vi "testVI.vi"() -> ()   [LabVIEW 2015]
panel:
  out "Remote Call":bool
  out "result string":string
  out "VI Path 2":path
  out "call chain":string[](array[string])
  out "VI Path":path
  out "Is Clone VI":bool
  out "Is In Packed Library":bool
  out "Is Instance":bool
  out "Is Probe":bool
  out "Callers' Names":string[](array[string])
  out "Execution:Preferred Exec System":T1(ring)
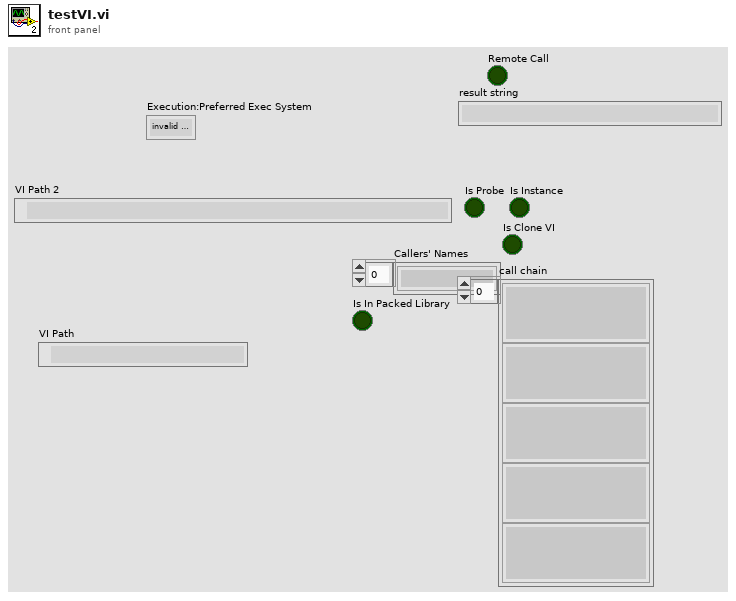
[diagram p1: front panel]
types:
  T1 = enum32{"invalid execution system", "user interface", "standard", "instrument i/o", "data acquisition", "other 1", "other 2", "same as caller"}
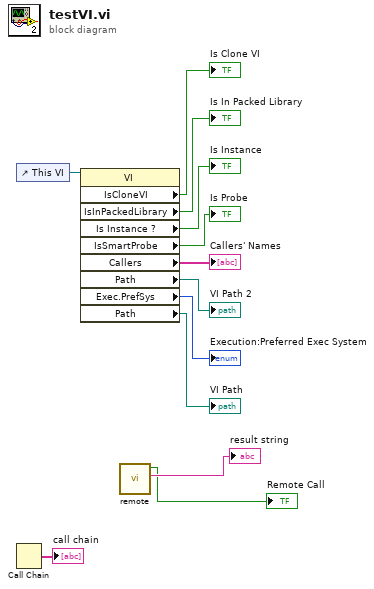
[diagram p0: block diagram]
diagram:
  n1 = Call Chain() -> (call chain=→"call chain":string[])
  n2 = control-ref of="This VI"() -> (w12:refnum<vi>)
  n3 = property class="VI"(reference=w12) -> ("IsCloneVI"=→"Is Clone VI":bool, "IsInPackedLibrary"=→"Is In Packed Library":bool, "Is Instance ?"=→"Is Instance":bool, "IsSmartProbe"=→"Is Probe":bool, "Callers"=→"Callers' Names":string[], "Path"=→"VI Path 2":path, "Exec.PrefSys"=→"Execution:Preferred Exec System":T1, "Path"=→"VI Path":path)  [unwired: 1 in, 2 out]
  n4 = call "remote.vi"() -> ("Caller string"=→"result string":string, "Remote Call"=→"Remote Call":bool)  [unwired: 9 in, 1 out]
